vi "SetFlySettings_USB7855R.vi"(9 "output cluster 3":T1, 11 "FPGA VI Reference Out":refnum<k20>) -> ()   [LabVIEW 2023]
uses:
  <vilib>/Utility/error.llb/Error Cluster From Error Code.vi
  <vilib>/rvi/errors/niLvFpgaAdjustHostInterfaceError.vi
  <vilib>/rvi/interface/nirviReadWriteControl/nirviReadWriteControl.xnode
  NiFpgaLv.dll
  <vilib>/rvi/interface/Simulation/niFpgaSimulationCallBeginRW.vi
panel:
  out "Fly Cluster":T2 {"Value" format="%.32g"}
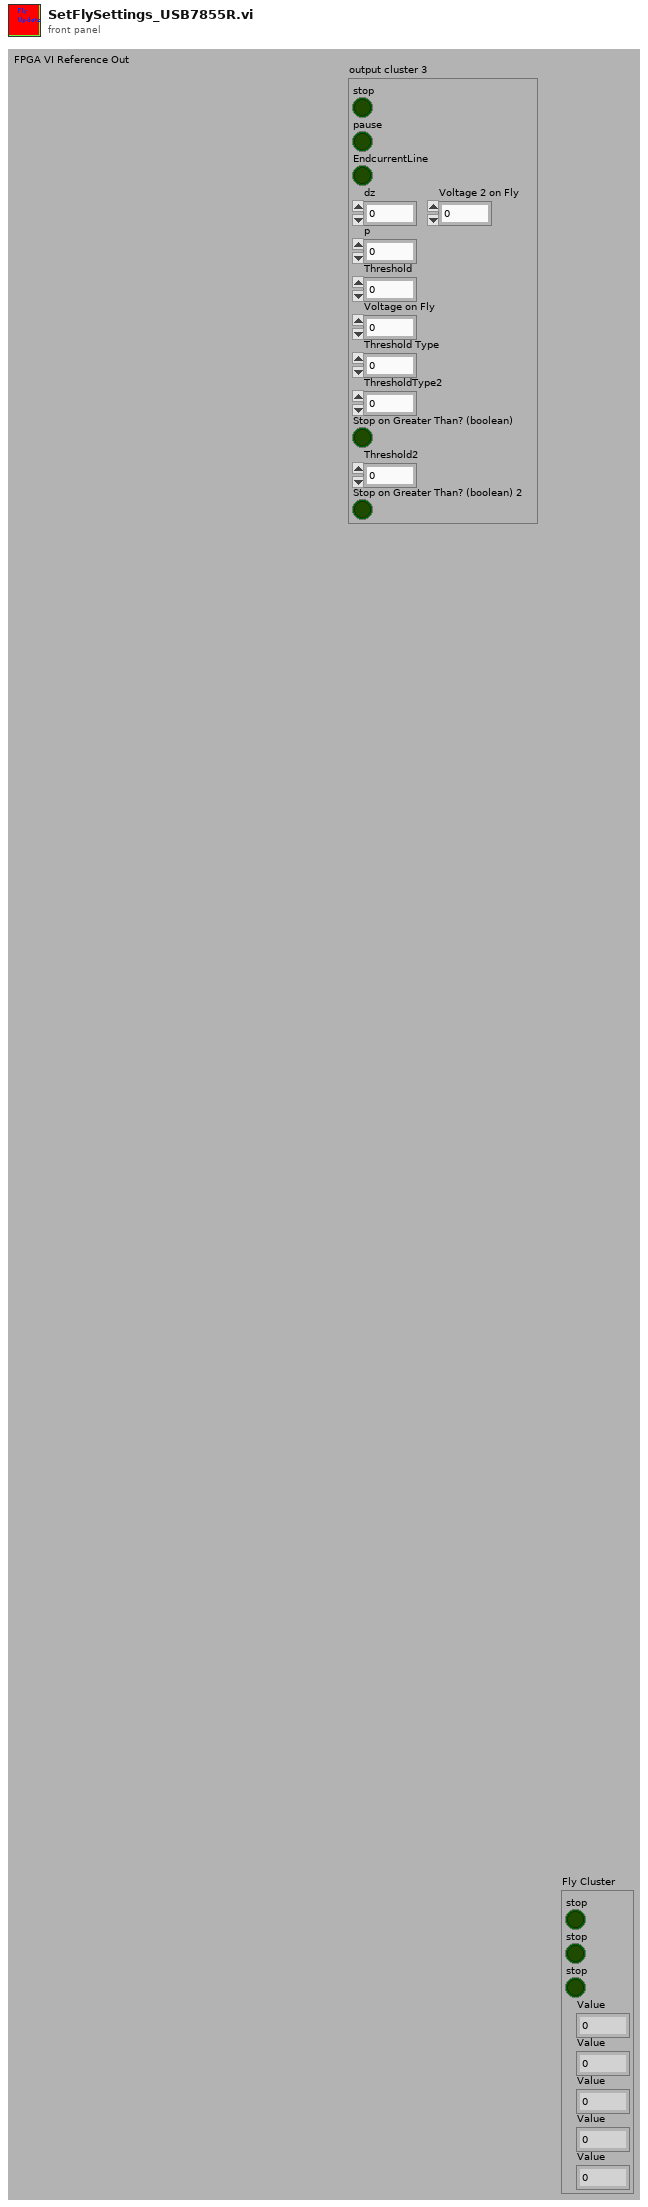
[diagram p1: front panel]
types:
  T1 = cluster{"stop":bool, "pause":bool, "EndcurrentLine":bool, "dz":i32, "p":fxp<+/-,32,1>, "Threshold":i32, "Voltage on Fly":i16, "Threshold Type":u8, "ThresholdType2":u8, "Stop on Greater Than? (boolean)":bool, "Threshold2":i32, "Stop on Greater Than? (boolean) 2":bool, "Voltage 2 on Fly":i16}
  T2 = cluster{"stop":bool, "stop":bool, "stop":bool, "Value":i32, "Value":fxp<+/-,32,1>, "Value":i32, "Value":i32, "Value":i32}
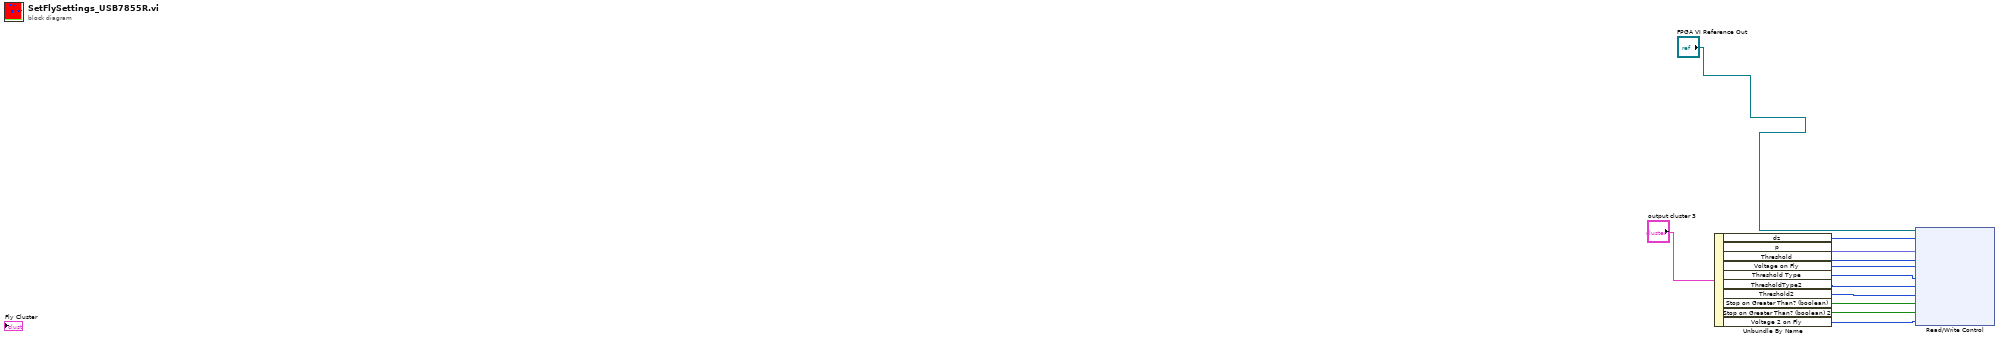
[diagram p0: block diagram]
diagram:
  n1 = Unbundle By Name("output cluster 3") -> ("dz"=w8:i32, "p"=w11:fxp<+/-,32,1>, "Threshold"=w12:i32, "Voltage on Fly"=w10:i16, "Threshold Type"=w9:u8, "ThresholdType2"=w6:u8, "Threshold2"=w5:i32, "Stop on Greater Than? (boolean)"=w4:bool, "Stop on Greater Than? (boolean) 2"=w3:bool, "Voltage 2 on Fly"=w2:i16)
  n2 = xnode "Read/Write Control"("FPGA VI Reference In"="FPGA VI Reference Out", "Upper limit Of dZ"=w8, "P"=w11, "Feedback_Threshold"=w12, "V on Fly"=w10, "FeedBackType"=w9, "FeedBackType 2"=w6, "Feedback_Threshold 2"=w5, "GreaterThan"=w4, "GreaterThan 2"=w3, "V2 on Fly"=w2) -> ()  [unwired: 1 in, 2 out]
